vi "Explode.vi"(11 "Asteroid in":refnum<class "Planet.lvclass">) -> (3 "Asteroid out":refnum<class "Planet.lvclass">)   [LabVIEW 2015]
uses:
  Planet.lvclass
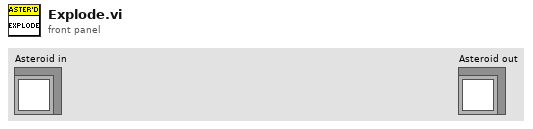
[diagram p1: front panel]
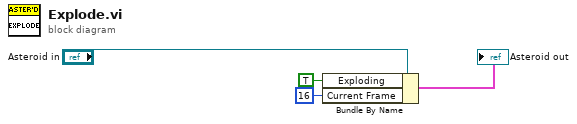
[diagram p0: block diagram]
diagram:
  n1 = Bundle By Name(cluster="Asteroid in", "Exploding"=TRUE, "Current Frame"=16) -> (→"Asteroid out":cluster{})
